vi "polcal.vi"(9 "file path (dialog if empty)":path, 10 "BuffNr":i16, 11 "ph":u64) -> (3 "hout":u64)   [LabVIEW 2014]
uses:
  <vilib>/Platform/TimedLoop/XDataNode/timing_clust.ctl
  <vilib>/Platform/TimedLoop/XDataNode/nitl_modes.ctl
  <vilib>/Platform/TimedLoop/XDataNode/wakeup.ctl
  gfitsio/cfitsio-bitpix.ctl
  <vilib>/platform/TimedLoop/XDataNode/XDataNode.xnode
  <userlib>/Newport ESP301/Newport ESP301.lvlib
  <vilib>/Platform/TimedLoop/XDataNode/XDNodeRunTimeDep.lvlib
  gfitsio/gfitsio.lvlib
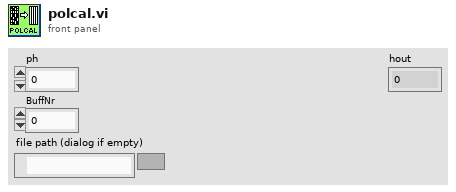
[diagram p1: front panel]
types:
  T1 = enum16{"Find +0 Position Count", "Find Home and Index Signals", "Find Home Signal", "Find Positive Limit Signal", "Find Negative Limit Signal", "Find Positve Limit and Index Signals", "Find Negative Limit and Index Signals"}
  T2 = typedef "XDNodeRunTimeDep.lvlib/timing_clust.ctl" = cluster{"Expected End [f-1]":u64, "Actual End [f-1]":u64, "Finished Late? [f-1]":bool, "Expected End [i-1]":u64, "Actual End [i-1]":u64, "Finished Late? [i-1]":bool, "Expected Start [i]":u64, "Actual Start [i]":u64, "Expected Start [f]":u64, "Actual Start [f]":u64, "Source Name":string, "Structure Name":string, "Period":i64, "Deadline":i64, "Offset":i64, "Start":i64, "Priority":i32, "Timeout":i32, "Mode":T3, "Wakeup Reason":T4, "Error":errorcluster, "Source Type":string, "Secondary Source Type":string, "Global End Time":u64, "Global Start Time":u64, "Frame Duration":u64, "Iteration Duration":u64, "Assigned CPU":i32, "I/O Scan Engine Mode":u32}
  T3 = typedef "XDNodeRunTimeDep.lvlib/nitl_modes.ctl" = enum32{"No Change", "Process missed periods, maintain original phase", "Discard missed periods, maintain original phase", "Process missed periods, ignore original phase", "Discard missed periods, ignore original phase"}
  T4 = typedef "XDNodeRunTimeDep.lvlib/wakeup.ctl" = enum32{"Normal", "Aborted", "Asynchronous wakeup", "Timing source error", "Timed loop error", "Timeout"}
  T5 = enum16{"open", "open or create", "create or replace", "create", "open (read only)"}
  T6 = typedef "gfitsio.lvlib/cfitsio-bitpix.ctl" = i32
  T7 = typedef "gfitsio.lvlib/gfitsio-refnum.ctl" = refnum<k1>
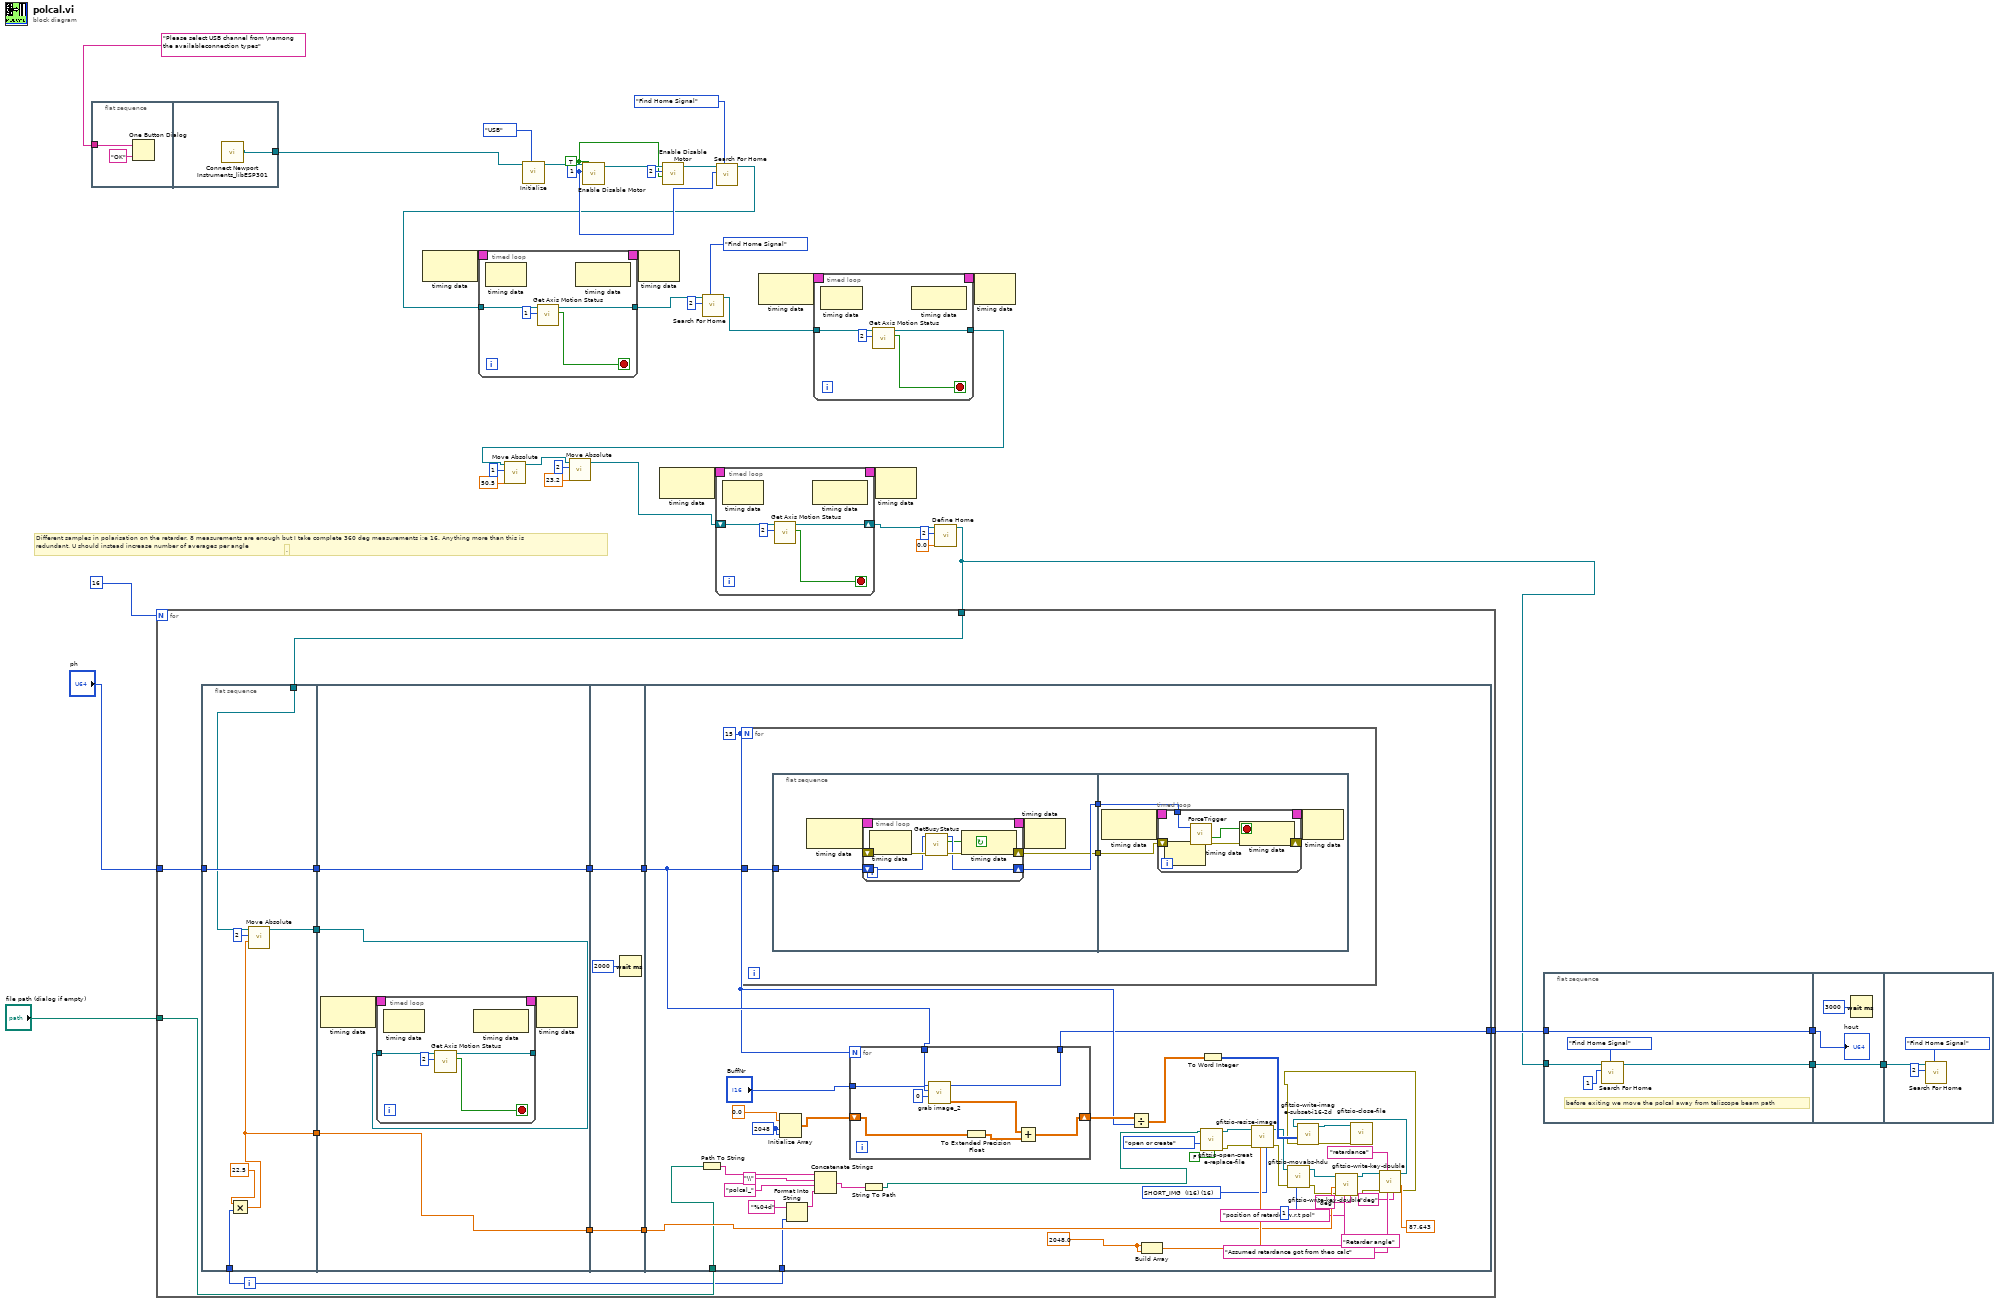
[diagram p0: block diagram]
diagram:
  w35 = TRUE ("Action (F - OFF)")
  w32 = 1 ("Axis (1)")
  # "."
  # "Different samples in polarisation on the retarder. 8 measurements are enough but I take complete 360 deg measurements i;e 16. Anything more than this is \nredundant. U should instead increase number of averages per angle"
  n1 = flat-sequence {
    tunnel: "Please select USB channel from \namong the availableconnection types" ("message") -> [w41]
    tunnel: [w42] -> w10
    frame #0 {
      n2 = One Button Dialog(message=w41, button name ("OK")="OK") -> ()  [unwired: 1 out]
    }
    frame #1 {
      n3 = call <userlib>:"Connect Newport Instruments_libESP301.vi"() -> ("VISA resource name (duplicate)"=w42:refnum<visa-resource-name>)  [unwired: 7 in, 4 out]
    }
  }
  n4 = node-c288() -> (w31:T2)  [unwired: 1 in]
  n5 = call <userlib>:"Initialize.vi"("VISA resource name"=w10, "Serial Link (RS232)"=enum16{"RS232", "USB"}."USB") -> ("VISA resource name out"=w38:refnum<visa-resource-name>)  [unwired: 7 in, 1 out]
  n6 = call <userlib>:"Enable Disable Motor.vi"("Action (F - OFF)"=w35, "Axis (1)"=w32, "VISA resource name"=w38) -> ("VISA resource name out"=w37:refnum<visa-resource-name>)  [unwired: 3 in, 1 out]
  n7 = node-c288() -> (w20:T2)  [unwired: 1 in]
  n8 = call <userlib>:"Enable Disable Motor.vi"("Action (F - OFF)"=w35, "Axis (1)"=2, "VISA resource name"=w37) -> ("VISA resource name out"=w34:refnum<visa-resource-name>)  [unwired: 3 in, 1 out]
  n9 = call <userlib>:"Search For Home.vi"("Home mode"=T1."Find Home Signal", "Axis (1)"=w32, "VISA resource name"=w34) -> ("VISA resource name out"=w29:refnum<visa-resource-name>)  [unwired: 4 in, 1 out]
  n10 = timed-loop {
    timing: w31 -> [_]
    timing-out: [_] -> w30
    tunnel: w29 -> [w45]
    tunnel: [w43] -> w28
    stop <- w46 stop-if-true
    n11 = node-c288() -> ()  [unwired: 1 in, 1 out]
    n12 = call <userlib>:"Get Axis Motion Status.vi"("Axis (1)"=1, "VISA resource name"=w45) -> ("Motion Done"=w46:bool, "VISA resource name out"=w43:refnum<visa-resource-name>)  [unwired: 3 in, 1 out]
    n13 = node-c288() -> ()  [unwired: 1 in, 1 out]
  }
  n14 = node-c288(w30) -> ()  [unwired: 1 out]
  n15 = call <userlib>:"Search For Home.vi"("Home mode"=T1."Find Home Signal", "Axis (1)"=2, "VISA resource name"=w28) -> ("VISA resource name out"=w23:refnum<visa-resource-name>)  [unwired: 4 in, 1 out]
  n16 = node-c288() -> (w25:T2)  [unwired: 1 in]
  n17 = timed-loop {
    timing: w25 -> [_]
    timing-out: [_] -> w24
    tunnel: w23 -> [w51]
    tunnel: [w49] -> w7
    stop <- w52 stop-if-true
    n18 = node-c288() -> ()  [unwired: 1 in, 1 out]
    n19 = call <userlib>:"Get Axis Motion Status.vi"("Axis (1)"=2, "VISA resource name"=w51) -> ("Motion Done"=w52:bool, "VISA resource name out"=w49:refnum<visa-resource-name>)  [unwired: 3 in, 1 out]
    n20 = node-c288() -> ()  [unwired: 1 in, 1 out]
  }
  n21 = call <userlib>:"Move Absolute.vi"("Position (0 units)"=50.5, "Axis (1)"=1, "VISA resource name"=w7) -> ("VISA resource name out"=w4:refnum<visa-resource-name>)  [unwired: 3 in, 1 out]
  n22 = call <userlib>:"Move Absolute.vi"("Position (0 units)"=23.2, "Axis (1)"=2, "VISA resource name"=w4) -> ("VISA resource name out"=w18:refnum<visa-resource-name>)  [unwired: 3 in, 1 out]
  n23 = timed-loop {
    timing: w20 -> [_]
    timing-out: [_] -> w19
    shift-right: [w55] -> w16
    shift-left: w18 -> [w57]
    stop <- w58 stop-if-true
    n24 = node-c288() -> ()  [unwired: 1 in, 1 out]
    n25 = call <userlib>:"Get Axis Motion Status.vi"("Axis (1)"=2, "VISA resource name"=w57) -> ("Motion Done"=w58:bool, "VISA resource name out"=w55:refnum<visa-resource-name>)  [unwired: 3 in, 1 out]
    n26 = node-c288() -> ()  [unwired: 1 in, 1 out]
  }
  n27 = node-c288(w19) -> ()  [unwired: 1 out]
  n28 = call <userlib>:"Define Home.vi"("Home Position (0 units)"=0.0, "Axis (1)"=2, "VISA resource name"=w16) -> ("VISA resource name out"=w8:refnum<visa-resource-name>)  [unwired: 3 in, 1 out]
  n29 = for {
    N: 16 -> [_]
    tunnel: "ph" -> [w72]
    tunnel: "file path (dialog if empty)" -> [w63]
    tunnel: w8 -> [w70]
    tunnel: [w61] -> w9
    i -> [w62]
    n30 = flat-sequence {
      tunnel: w72 -> [w79]
      tunnel: [w79] -> w71
      tunnel: w70 -> [w78]
      tunnel: w62 -> [w76]
      tunnel: [w74] -> w67
      tunnel: [w73] -> w66
      tunnel: w71 -> [w84]
      tunnel: [w84] -> w69
      tunnel: w67 -> [w81]
      tunnel: w66 -> [w80]
      tunnel: [w80] -> w64
      tunnel: w69 -> [w95]
      tunnel: [w95] -> w68
      tunnel: [w93] -> w65
      tunnel: w64 -> [w93]
      tunnel: w68 -> [w135]
      tunnel: w65 -> [w117]
      tunnel: w63 -> [w106]
      tunnel: w62 -> [w102]
      tunnel: [w96] -> w61
      frame #0 {
        n31 = Multiply(x=22.5, y=w76) -> (x*y=w73:dbl)
        n32 = call <userlib>:"Move Absolute.vi"("Position (0 units)"=w73, "Axis (1)"=2, "VISA resource name"=w78) -> ("VISA resource name out"=w74:refnum<visa-resource-name>)  [unwired: 3 in, 1 out]
      }
      frame #1 {
        n33 = node-c288() -> (w83:T2)  [unwired: 1 in]
        n34 = timed-loop {
          timing: w83 -> [_]
          timing-out: [_] -> w82
          tunnel: w81 -> [w87]
          tunnel: [w85] -> _
          stop <- w88 stop-if-true
          n35 = node-c288() -> ()  [unwired: 1 in, 1 out]
          n36 = call <userlib>:"Get Axis Motion Status.vi"("Axis (1)"=2, "VISA resource name"=w87) -> ("Motion Done"=w88:bool, "VISA resource name out"=w85:refnum<visa-resource-name>)  [unwired: 3 in, 1 out]
          n37 = node-c288() -> ()  [unwired: 1 in, 1 out]
        }
        n38 = node-c288(w82) -> ()  [unwired: 1 out]
      }
      frame #2 {
        n39 = Wait (ms)(milliseconds to wait=u32 2000) -> ()  [unwired: 1 out]
      }
      frame #3 {
        w131 = T6 16 items=["<invalid type>"=0, "BYTE_IMG  (U8)"=8, "SHORT_IMG  (I16)"=16, "USHORT_IMG  (U16)"=20, "LONG_IMG  (I32)"=32, "ULONG_IMG  (U32)"=40, "FLOAT_IMG  (SGL)"=-32, "DOUBLE_IMG  (DBL)"=-64] ("image data type")
        w133 = 2048.0 ("element")
        w138 = 2048 ("dimension size")
        w123 = 15
        n40 = Path To String(path=w106) -> (string=w105:string)
        n41 = for {
          N: w123 -> [_]
          tunnel: w135 -> [w149]
          n42 = flat-sequence {
            tunnel: [w154] -> w151
            tunnel: [w153] -> w150
            tunnel: w149 -> [w152]
            tunnel: w151 -> [w167]
            tunnel: w150 -> [w166]
            frame #0 {
              n43 = node-c288() -> (w156:T2)  [unwired: 1 in]
              n44 = timed-loop {
                shift-right: [w159] -> w154
                shift-left: w152 -> [w157]
                shift-right: [w160] -> w153
                shift-left: _ -> [w161]
                timing: w156 -> [_]
                timing-out: [_] -> w155
                stop <- w158 continue-if-true
                n45 = node-c288() -> ()  [unwired: 1 in, 1 out]
                n46 = call <userlib>:"GetBusyStatus.vi"("error in (no error)"=w161, "ph"=w157) -> ("error out"=w160:errorcluster, "BusyState"=w158:bool, "hout"=w159:u64)  [unwired: 2 in, 1 out]
                n47 = node-c288() -> ()  [unwired: 1 in, 1 out]
              }
              n48 = node-c288(w155) -> ()  [unwired: 1 out]
            }
            frame #1 {
              n49 = node-c288() -> (w169:T2)  [unwired: 1 in]
              n50 = timed-loop {
                shift-right: [w171] -> _
                shift-left: w166 -> [w172]
                timing: w169 -> [_]
                timing-out: [_] -> w168
                tunnel: w167 -> [w170]
                stop <- w173 stop-if-true
                n51 = node-c288() -> ()  [unwired: 1 in, 1 out]
                n52 = call <userlib>:"ForceTrigger.vi"("ph"=w170, "error in (no error)"=w172) -> ("Triggered"=w173:bool, "error out"=w171:errorcluster)  [unwired: 1 in, 2 out]
                n53 = node-c288() -> ()  [unwired: 1 in, 1 out]
              }
              n54 = node-c288(w168) -> ()  [unwired: 1 out]
            }
          }
        }
        n55 = Initialize Array(0.0 ("element"), w138, w138) -> (w139:dbl[][])
        n56 = Format Into String(format string="%04d", w102) -> (resulting string=w100:string)  [unwired: 2 in, 1 out]
        n57 = Concatenate Strings(w105, "\\" ("string"), "polcal_" ("string"), w100) -> (w99:string)
        n58 = for {
          N: w123 -> [_]
          tunnel: "BuffNr" -> [w147]
          tunnel: w135 -> [w146]
          shift-right: [w142] -> w136
          shift-left: w139 -> [w145]
          tunnel: [w141] -> w96
          n59 = call "grab image_2.vi"("Image number"=u32 0, "BuffNr"=w147, "ph"=w146) -> ("output image"=w143:dbl[][], "hout"=w141:u64)  [unwired: 5 in, 2 out]
          n60 = To Extended Precision Float(1:w145) -> (0:w144:ext[][])
          n61 = Add(x=w143, y=w144) -> (x+y=w142:ext[][])
        }
        n62 = String To Path(string=w99) -> (path=w98:path)
        n63 = Divide(x=w136, y=w123) -> (x/y=w127:ext[][])
        n64 = Build Array(w133, w133) -> (w132:dbl[])
        n65 = call "gfitsio-open-create-replace-file.vi"("advisory dialog? (display:T)"=FALSE, "function (open)"=T5."open or create", "file path (dialog if empty)"=w98) -> ("error out"=w128:errorcluster, "gfits refnum"=w134:T7)  [unwired: 6 in, 1 out]
        n66 = To Word Integer(number=w127) -> (16bit integer=w126:i16[][])
        n67 = call "gfitsio-resize-image.vi"("image data type"=w131, "naxes"=w132, "error in (no error)"=w128, "gfits refnum"=w134) -> ("error out"=w121:errorcluster, "dup gfits refnum"=w122:T7)  [unwired: 6 in]
        n68 = call "gfitsio-movabs-hdu.vi"("hdunum"=1, "error in (no error)"=w121, "gfits refnum"=w122) -> ("error out"=w109:errorcluster, "dup gfits refnum"=w119:T7)  [unwired: 6 in, 1 out]
        n69 = call "gfitsio-write-key-double.vi"("units"="deg", "comment"="position of retarder w.r.t pol", "keyname"="Retarder angle", "error in (no error)"=w109, "value"=w117, "gfits refnum"=w119) -> ("error out"=w108:errorcluster, "dup gfits refnum"=w115:T7)  [unwired: 4 in]
        n70 = call "gfitsio-write-key-double.vi"("units"="deg", "comment"="Assumed retardance got from theo calc", "keyname"="retardance", "error in (no error)"=w108, "value"=87.643, "gfits refnum"=w115) -> ("error out"=w107:errorcluster, "dup gfits refnum"=w110:T7)  [unwired: 4 in]
        n71 = call "gfitsio-write-image-subset-i16-2d.vi"("error in (no error)"=w107, "data"=w126, "gfits refnum"=w110) -> ("error out"=w124:errorcluster, "dup gfits refnum"=w125:T7)  [unwired: 7 in]
        n72 = call "gfitsio-close-file.vi"("error in (no error)"=w124, "gfits refnum"=w125) -> ()  [unwired: 8 in, 2 out]
      }
    }
  }
  n73 = node-c288(w24) -> ()  [unwired: 1 out]
  n74 = flat-sequence {
    tunnel: w9 -> [w182]
    tunnel: w8 -> [w180]
    tunnel: [w182] -> w3
    tunnel: [w178] -> w2
    tunnel: w3 -> [w183]
    tunnel: w2 -> [w185]
    tunnel: [w185] -> w1
    tunnel: w1 -> [w188]
    frame #0 {
      # "before exiting we move the polcal away from teliscope beam path"
      n75 = call <userlib>:"Search For Home.vi"("Home mode"=T1."Find Home Signal", "Axis (1)"=1, "VISA resource name"=w180) -> ("VISA resource name out"=w178:refnum<visa-resource-name>)  [unwired: 4 in, 1 out]
    }
    frame #1 {
      n76 = Wait (ms)(milliseconds to wait=u32 3000) -> ()  [unwired: 1 out]
      "hout" <- w183
    }
    frame #2 {
      n77 = call <userlib>:"Search For Home.vi"("Home mode"=T1."Find Home Signal", "Axis (1)"=2, "VISA resource name"=w188) -> ()  [unwired: 4 in, 2 out]
    }
  }
